vi "LEDDebugColorSwerve.vi"(1 "Azimuth_Angle (deg [-180,180])":dbl, 2 "Drive Velocity (ft/s)":dbl) -> (0 "Color":u32(colorbox))   [LabVIEW 2020]
doc: "Sets the LED hue based on the swerve azimuth angle and the intensity based on the swerve drive speed."
uses:
  <vilib>/vision/NI_Vision_Development_Module.lvlib
  GlobalDrivebase.vi
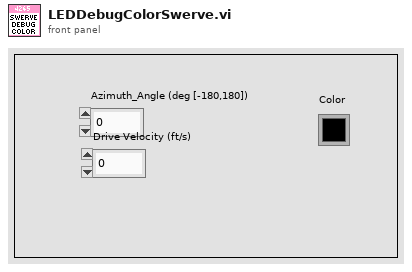
[diagram p1: front panel]
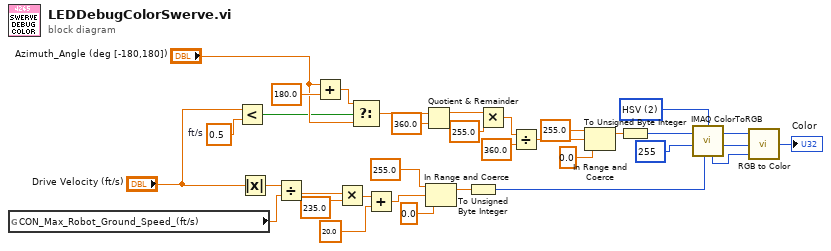
[diagram p0: block diagram]
diagram:
  w4 = 0.5  # ft/s
  w34 = u16 2 items=["RGB", "HSL", "HSV", "HSI"] ("Color Mode")
  n1 = global read "GlobalDrivebase.vi" "CON_Max_Robot_Ground_Speed_(ft/s)"() -> (w1:dbl)
  n2 = Less?(x="Drive Velocity (ft/s)", y=w4) -> (x < y?=w6:bool)
  n3 = Absolute Value(x="Drive Velocity (ft/s)") -> (abs(x)=w25:dbl)
  n4 = Divide(x=w25, y=w1) -> (x/y=w30:dbl)
  n5 = Add(x="Azimuth_Angle (deg [-180,180])", y=180.0) -> (x+y=w21:dbl)
  n6 = Multiply(x=w30, y=235.0) -> (x*y=w7:dbl)
  n7 = Select(t=w21, s=w6, f="Azimuth_Angle (deg [-180,180])") -> (s? t:f=w20:dbl)
  n8 = Add(x=w7, y=20.0) -> (x+y=w9:dbl)
  n9 = Quotient & Remainder(x=w20, y=360.0) -> (x-y*floor(x/y)=w18:dbl)  [unwired: 1 out]
  n10 = In Range and Coerce(upper limit=255.0, x=w9, lower limit=0.0) -> (coerced(x)=w26:dbl)  [unwired: 1 out]
  n11 = To Unsigned Byte Integer(number=w26) -> (unsigned 8bit integer=w2:u8)
  n12 = Multiply(x=w18, y=255.0) -> (x*y=w17:dbl)
  n13 = Divide(x=w17, y=360.0) -> (x/y=w14:dbl)
  n14 = In Range and Coerce(upper limit=255.0, x=w14, lower limit=0.0) -> (coerced(x)=w13:dbl)  [unwired: 1 out]
  n15 = To Unsigned Byte Integer(number=w13) -> (unsigned 8bit integer=w12:u8)
  n16 = call "IMAQ ColorToRGB"("Green or Sat value"=u8 255, "Blue or Luma or Val or Inten value"=w2, "Red or Hue value"=w12, "Color Mode"=w34) -> ("Blue value"=w31:u8, "Green value"=w32:u8, "Red value"=w33:u8)  [unwired: 1 in, 1 out]
  n17 = call <vilib>:"RGB to Color.vi"("B"=w31, "G"=w32, "R"=w33) -> ("Color"=→"Color":u32)
